vi "Decorator.vi"(10 "jettl":refnum<class "jettl.lvclass">, 11 "TEMPLATE jettl in":refnum<class "TEMPLATE jettl.lvclass">) -> (3 "TEMPLATE jettl out":refnum<class "TEMPLATE jettl.lvclass">)   [LabVIEW 2021, in "_Template.lvlib" / "Templates.lvlib" / "TEMPLATE jettl.lvlib" / "TEMPLATE jettl.lvclass"]
uses:
  TEMPLATE jettl.lvclass
  TEMPLATE jettl.lvclass/TEMPLATE jettl.ctl
  jettl/jettl/jettl/jettl.lvclass
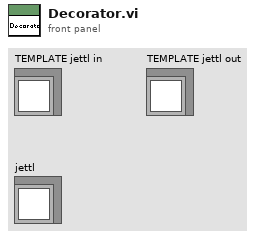
[diagram p1: front panel]
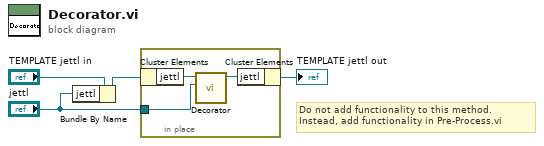
[diagram p0: block diagram]
diagram:
  # "Do not add functionality to this method. Instead, add functionality in Pre-Process.vi"
  n1 = Bundle By Name(cluster="TEMPLATE jettl in", "jettl"="jettl") -> (w3:refnum<class "TEMPLATE jettl.lvclass">)
  n2 = in-place {
    in-place-border: "jettl" -> [w5]
    n3 = in-place-cluster #1(w3) -> ("jettl"=w7:refnum<class "jettl.lvclass">)
    n4 = call-dynamic "Decorator.vi"("jettl"=w5, "jettl in"=w7) -> ("jettl out"=w6:refnum<class "jettl.lvclass">)  [unwired: 9 in]
    n5 = in-place-cluster #1("jettl"=w6) -> (→"TEMPLATE jettl out":refnum<class "TEMPLATE jettl.lvclass">)
  }
